vi "Therapy.vi"(0 "Theraputic Freq (MHz)":dbl=0.10000000000000009 min=0.0001 max=250.0 format="%.3f", 1 "ExitSendCmd":bool, 2 "Time on":dbl=1.0 format="%.5f", 3 "Therapy amplitude (mV)":dbl=50.0 min=10.0 max=1000.0 format="%.2f", 4 "SkipInitValues?":bool, 5 "start scan":bool) -> ()   [LabVIEW 2022 SP3]
uses:
  Motion Controllers/-MotionRoutines/MotionGlobals.vi
  <vilib>/DAQmx/create/channels.llb/DAQmx Create Channel (CO-Pulse Generation-Time).vi
  Pulsers/PulserGlobals.vi
panel:
  in  "VISA session":refnum<visa-resource-name>
  in  "Emergency stop":bool
  # "Pushing escape will also stop therapy"
  # "(s)"
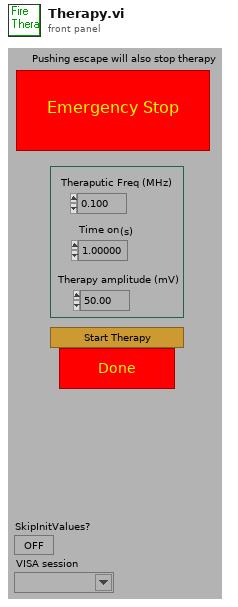
[diagram p1: front panel]
types:
  T1 = cluster{"Time on":dbl, "Theraputic Freq (MHz)":dbl, "Therapy amplitude (mV)":dbl}
  T2 = cluster{"Therapy frequency (MHz)":dbl, "Therapy amplitude (mV)":dbl, "time therapy on (s)":dbl, "Therapy Delay (ms) ":dbl, "Time (s)":dbl}
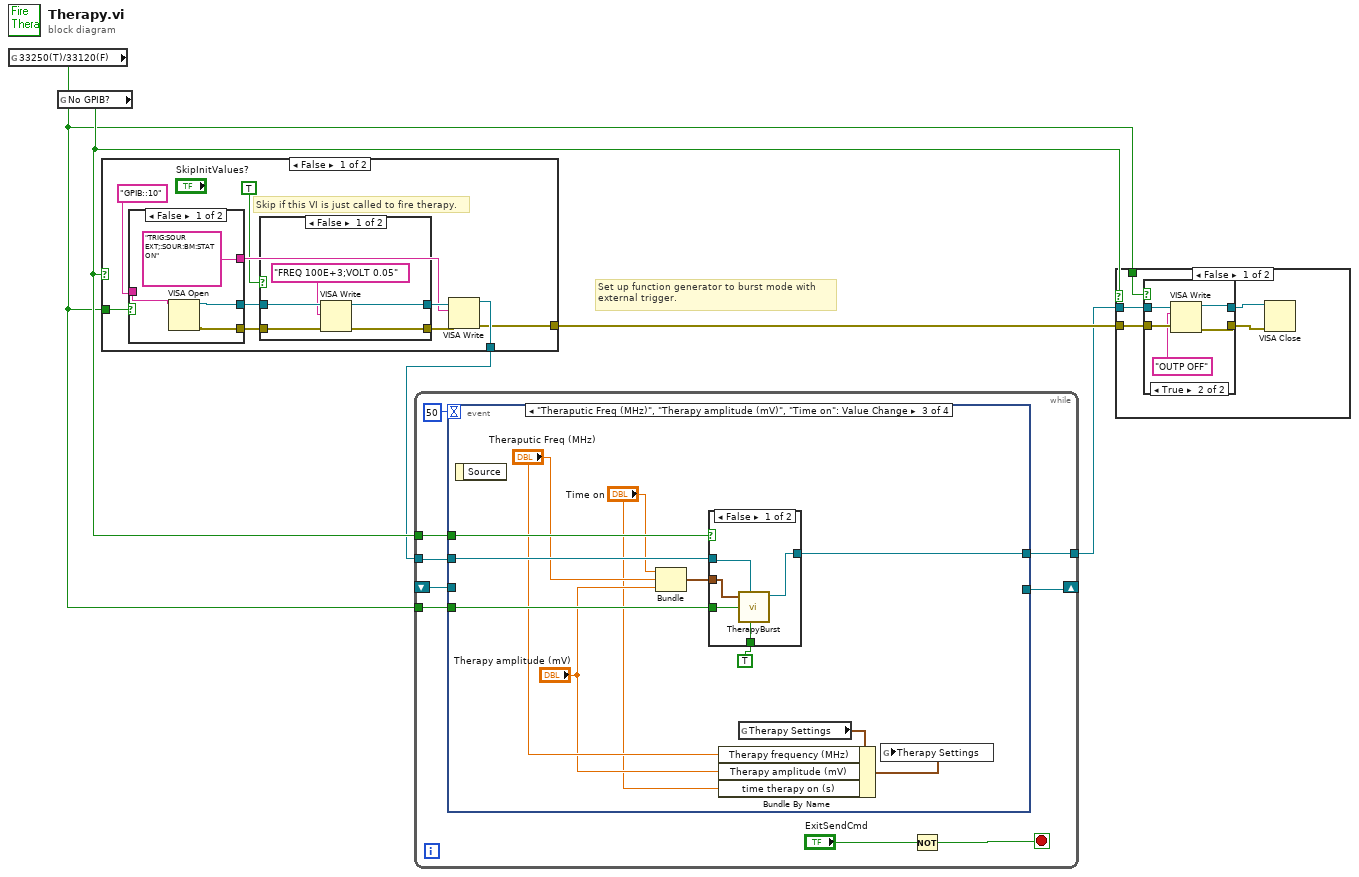
[diagram p0: block diagram]
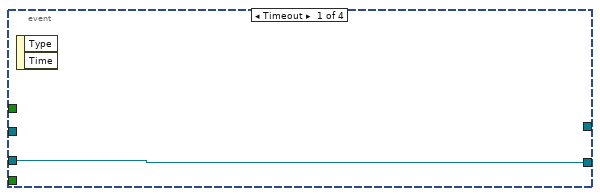
[diagram p2: hidden frame]
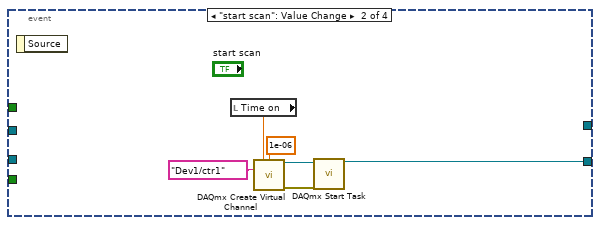
[diagram p3: hidden frame]
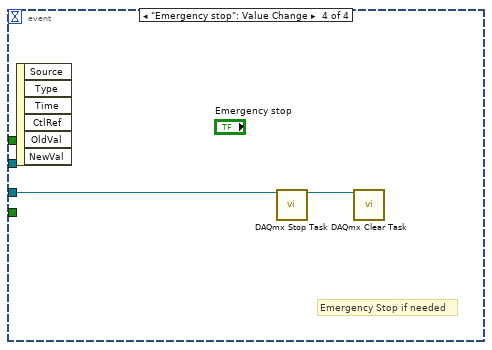
[diagram p5: hidden frame]
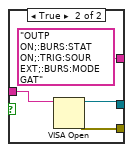
[diagram p8: hidden frame]
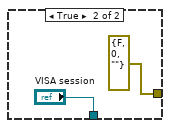
[diagram p10: hidden frame]
diagram:
  # "Set up function generator to burst mode with\nexternal trigger."
  n1 = global read "MotionGlobals.vi" "33250(T)/33120(F)"() -> (w3:bool)
  n2 = global read "MotionGlobals.vi" "No GPIB?"() -> (w4:bool)
  n3 = case shown="False" w4 {
    tunnel: [w15 "VISA session"] -> w2
    tunnel: [w14 errorcluster {"status"=FALSE, "code"=0, "source"=""} ("error out")] -> w5
    tunnel: w3 -> [w8 _]
    frame False {
      # "Skip if this VI is just called to fire therapy."
      n4 = case shown="False" w8 {
        tunnel: "GPIB::10" ("instrument descripter") -> [w16 w20]
        tunnel: [w18 w22] -> w12
        tunnel: [w17 w21] -> w11
        tunnel: ["TRIG:SOUR EXT;:SOUR:BM:STAT ON" "OUTP ON;:BURS:STAT ON;:TRIG:SOUR EXT;:BURS:MODE GAT"] -> w7
        frame False {
          n5 = VISA Open(VISA resource name=w16) -> (VISA resource name=w18:refnum<visa-resource-name>, error out=w17:errorcluster)  [unwired: 4 in]
        }
        frame True {
          n6 = VISA Open(VISA resource name=w20) -> (VISA resource name=w22:refnum<visa-resource-name>, error out=w21:errorcluster)  [unwired: 4 in]
        }
      }
      n7 = case shown="False" TRUE ("Case Constant\n(See Context Help)") {
        tunnel: w12 -> [w28 w30]
        tunnel: w11 -> [w27 w29]
        tunnel: [w26 w30] -> w10
        tunnel: [w25 w29] -> w9
        frame False {
          n8 = VISA Write(VISA resource name=w28, write buffer="FREQ 100E+3;VOLT 0.05", error in (no error)=w27) -> (VISA resource name out=w26:refnum<visa-resource-name>, error out=w25:errorcluster)  [unwired: 1 out]
        }
        frame True {
        }
      }
      n9 = VISA Write(VISA resource name=w10, write buffer=w7, error in (no error)=w9) -> (VISA resource name out=w15:refnum<visa-resource-name>, error out=w14:errorcluster)  [unwired: 1 out]
    }
    frame True {
    }
  }
  n10 = while {
    shift-right: [w41] -> _
    shift-left: _ -> [w40]
    tunnel: w4 -> [w37]
    tunnel: w3 -> [w36]
    tunnel: w2 -> [w35]
    tunnel: [w34] -> w1
    stop <- w38 stop-if-true
    n11 = event shown="[2] \"Theraputic Freq (MHz)\", \"Therapy amplitude (mV)\", \"Time on\": Value Change" {
      selector: _ -> [_ _ _ _]
      dyn-events: _ -> [_ _ _ _]
      timeout: 50 -> [_ _ _ _]
      tunnel: [w42 w44 _ _] -> w41
      tunnel: w40 -> [w42 _ _ w67]
      tunnel: w37 -> [_ _ w57 _]
      tunnel: w36 -> [_ _ w56 _]
      tunnel: w35 -> [_ _ w55 _]
      tunnel: [_ _ w54 _] -> w34
      event Timeout {
        n12 = event-data() -> ()  [unwired: 3 out]
      }
      event "start scan": Value Change {
        n13 = event-data() -> ()  [unwired: 2 out]
        n14 = local read "Time on"() -> (w43:dbl)
        n15 = call-poly <vilib>:"DAQmx Create Virtual Channel.vi"("high time"=w43, "low time"=1e-06, "counter"=tag "Dev1/ctr1") -> ("task out"=w48:refnum<k21>, "error out"=w47:errorcluster)  [unwired: 6 in, 5 out]
        n16 = call <vilib>:"DAQmx Start Task.vi"("task/channels in"=w48, "error in"=w47) -> ("task out"=w44:refnum<k21>)  [unwired: 13 out]
      }
      event "Theraputic Freq (MHz)", "Therapy amplitude (mV)", "Time on": Value Change {
        n17 = event-data() -> ()  [unwired: 2 out]
        n18 = Bundle("Time on"="Time on", "Theraputic Freq (MHz)"="Theraputic Freq (MHz)", "Therapy amplitude (mV)"="Therapy amplitude (mV)") -> (w59:T1)  [unwired: 1 out]
        n19 = case shown="False" w57 {
          tunnel: w59 -> [w64 _]
          tunnel: w55 -> [w63 w65]
          tunnel: [w61 w65] -> w54
          tunnel: TRUE ("Trigger (F) Gate(T)") -> [w60 _]
          tunnel: w56 -> [w62 _]
          frame False {
            n20 = call "TherapyBurst.vi"("Input Cluster"=w64, "VISA session in"=w63, "33250(T)/33120(F)"=w62, "Trigger (F) Gate(T)"=w60) -> ("VISA session out"=w61:refnum<visa-resource-name>)  [unwired: 2 in, 2 out]
          }
          frame True {
          }
        }
        n21 = global read "PulserGlobals.vi" "Therapy Settings"() -> (w53:T2)
        n22 = Bundle By Name(cluster=w53, "Therapy frequency (MHz)"="Theraputic Freq (MHz)", "Therapy amplitude (mV)"="Therapy amplitude (mV)", "time therapy on (s)"="Time on") -> (w52:T2)
        n23 = global write "PulserGlobals.vi" "Therapy Settings"(w52) -> ()
      }
      event "Emergency stop": Value Change {
        # "Emergency Stop if needed"
        n24 = event-data() -> ()  [unwired: 7 out]
        n25 = call <vilib>:"DAQmx Stop Task.vi"("task/channels in"=w67) -> ("task out"=w66:refnum<k21>)  [unwired: 1 in, 13 out]
        n26 = call <vilib>:"DAQmx Clear Task.vi"("task in"=w66) -> ()  [unwired: 1 in, 14 out]
      }
    }
    n27 = Not(x="ExitSendCmd") -> (.not. x?=w38:bool)
  }
  n28 = case shown="False" w4 {
    tunnel: w1 -> [w71 _]
    tunnel: w5 -> [w70 _]
    tunnel: w3 -> [w72 _]
    frame False {
      n29 = case shown="True" w72 {
        tunnel: [w74 w78] -> w69
        tunnel: w71 -> [w74 w76]
        tunnel: [w73 w79] -> w68
        tunnel: w70 -> [w73 w77]
        frame False {
        }
        frame True {
          n30 = VISA Write(VISA resource name=w76, write buffer="OUTP OFF", error in (no error)=w77) -> (VISA resource name out=w78:refnum<visa-resource-name>, error out=w79:errorcluster)  [unwired: 1 out]
        }
      }
      n31 = VISA Close(VISA resource name=w69, error in (no error)=w68) -> ()  [unwired: 1 out]
    }
    frame True {
    }
  }
